vi "Subvi AO mod.vi"(2 "AO channel":refnum<k21>="Connector1/AO0", 10 "Memory label":refnum<k21>="AO0 buffer") -> ()   [LabVIEW 2017]
uses:
  <vilib>/rvi/DataTransferAndStorage/Container/Common/niFpgaContainerExecOnDevCompGetState.vi
  <vilib>/rvi/Emulation/niFpgaEmulationIsFPGAContextNoSignature.vi
  <vilib>/rvi/DataTransferAndStorage/Container/Common/niFpgaContainerGetUniqueNameForEmu.vi
  <vilib>/rvi/Emulation/niFpgaProcessEmulError.vi
  <vilib>/rvi/Emulation/niFpgaSctlEmulationGetInTimedLoop.vi
  <vilib>/rvi/errors/nirviReportUnexpectedCaseInternalError (U32).vi
  <vilib>/rvi/Memory/Memory_Emulation/niFpgaMemoryEmulationCacheClearOnFirstRun.vi
  <vilib>/rvi/Memory/Memory_Emulation/nirvimemoryEmulationManagerCache_MakeExclusive.vi
  <vilib>/rvi/Memory/Memory_Emulation/niFpgaMemoryEmulationValidateCache.vi
  <vilib>/rvi/Memory/Memory_Emulation/nirvimemoryEmulationManagerCache_InsertValue.vi
  <vilib>/Utility/error.llb/Clear Errors.vi
  <vilib>/rvi/Memory/Memory_Emulation/nirvimemoryEmulationManagerCache_ReleaseExclusive.vi
  <vilib>/rvi/Memory/Memory_Emulation/nirvimemoryEmulationManagerCache_GetValue.vi
  <vilib>/rvi/Memory/Memory_Emulation/nirvimemoryEmulationManagerCache_SetValue.vi
  <vilib>/rvi/Emulation/niFpgaSctlEmulationResourceMgr.vi
  <vilib>/rvi/eio/common/nirviEmuTemplateMethod_errors.vi
  <vilib>/rvi/DataTransferAndStorage/Container/XNode/niFpgaContainer.xnode
  <vilib>/rvi/Memory/Memory_Emulation/niFpgaMemoryEmulationRefIn.vi
  <vilib>/eio/EIONode/EIONode.xnode
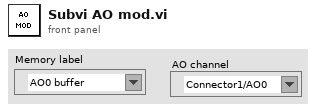
[diagram p1: front panel]
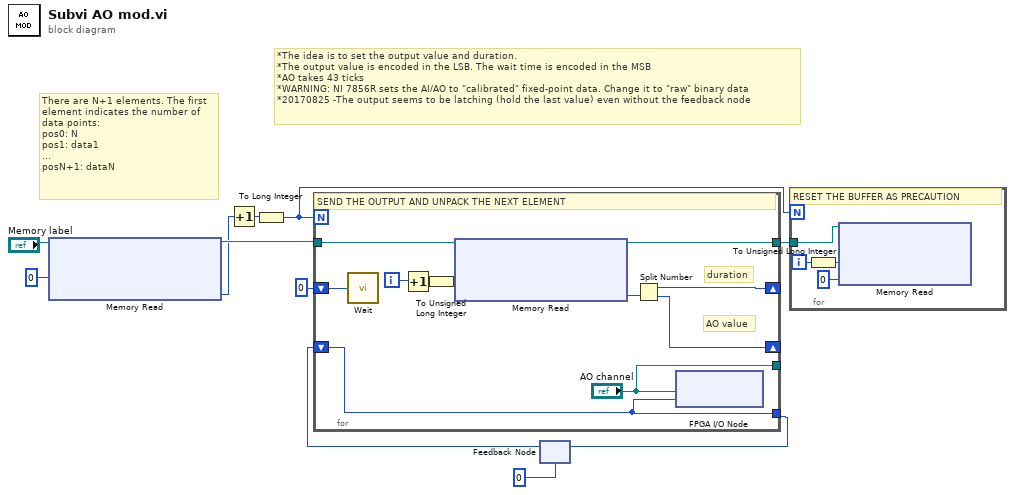
[diagram p0: block diagram]
diagram:
  # "There are N+1 elements. The first\nelement indicates the number of\ndata points:\npos0: N\npos1: data1\n...\nposN+1: dataN"
  # "*The idea is to set the output value and duration.\n*The output value is encoded in the LSB. The wait time is encoded in the MSB\n*AO takes 43 ticks\n*WARNING: NI 7856R sets the AI/AO to \"calibrated\" fixed-point data. Change it to \"raw\" binary data\n*20170825 -The output seems to be latching (hold the last value) even without the feedback node"
  n1 = xnode ("Memory Read")("Memory In"="Memory label", "Address"=u32 0) -> ("Memory Out"=w9:refnum<k21>, "Data"=w7:u32)
  n2 = Increment(x=w7) -> (x+1=w6:u32)
  n3 = To Long Integer(number=w6) -> (32bit integer=w5:i32)
  n4 = feedback #1(u16 0) -> (w4:u16)
  n5 = for {
    N: w5 -> [_]
    shift-right: [w21] -> _
    shift-left: u16 0 -> [w22]
    shift-right: [w19] -> _
    shift-left: w4 -> [w12]
    tunnel: ["AO channel"] -> _
    tunnel: [w18] -> w8
    tunnel: w9 -> [w16]
    tunnel: [w12] -> w2
    i -> [w15]
    # "duration"
    # "AO value"
    # "SEND THE OUTPUT AND UNPACK THE NEXT ELEMENT"
    n6 = call "Wait"("Count(Ticks)"=w22) -> ()  [unwired: 1 out]
    n7 = Increment(x=w15) -> (x+1=w14:i32)
    n8 = To Unsigned Long Integer(number=w14) -> (unsigned 32bit integer=w13:u32)
    n9 = xnode ("Memory Read")("Memory In"=w16, "Address"=w13) -> ("Memory Out"=w18:refnum<k21>, "Data"=w20:u32)
    n10 = Split Number(x=w20) -> (hi(x)=w21:u16, lo(x)=w19:u16)
    n11 = xnode "FPGA I/O Node"("I/O Item"=w12, "FPGA I/O In"="AO channel") -> ()  [unwired: 1 out]
  }
  n12 = feedback-in #1(w2) -> ()
  n13 = for {
    N: w5 -> [_]
    tunnel: w8 -> [w26]
    i -> [w24]
    # "RESET THE BUFFER AS PRECAUTION"
    n14 = To Unsigned Long Integer(number=w24) -> (unsigned 32bit integer=w23:u32)
    n15 = xnode ("Memory Read")("Address"=w23, "Data"=u32 0, "Memory In"=w26) -> ()  [unwired: 1 out]
  }
